vi "getConnectionPoints.vi"(0 "reference":refnum<class "SegmentedLineEdge.lvclass">, 5 "error in (no error)":errorcluster) -> (14 "reference out":refnum<class "SegmentedLineEdge.lvclass">, 15 "line":T1[](array[typedef]) {"y" format="%.2f"; "x" format="%.2f"}, 19 "error out":errorcluster)   [LabVIEW 2016, in "SegmentedLineEdge.lvclass"]
doc: "public Line2D getConnectionPoints()"
uses:
  <resource>/Framework/Providers/Open_GDS/UML/SegmentedLineEdge_class/SegmentedLineEdge.lvclass
  <resource>/Framework/Providers/Open_GDS/UML/General/Point/Point Point2D.ctl
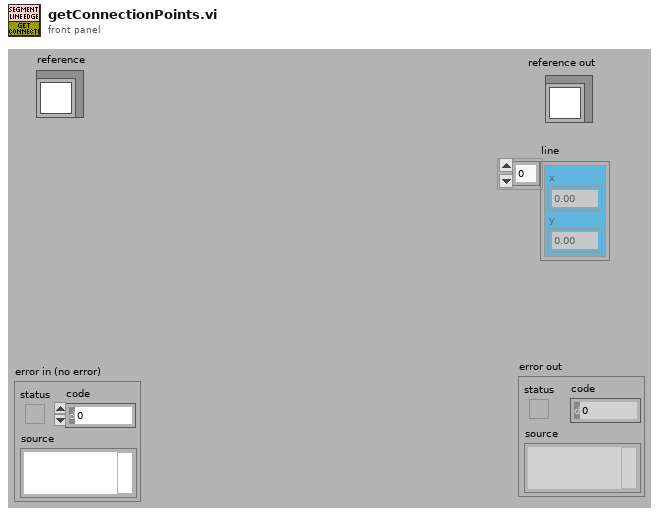
[diagram p1: front panel]
types:
  T1 = typedef "Point Point2D.ctl" = cluster{"x":dbl, "y":dbl}
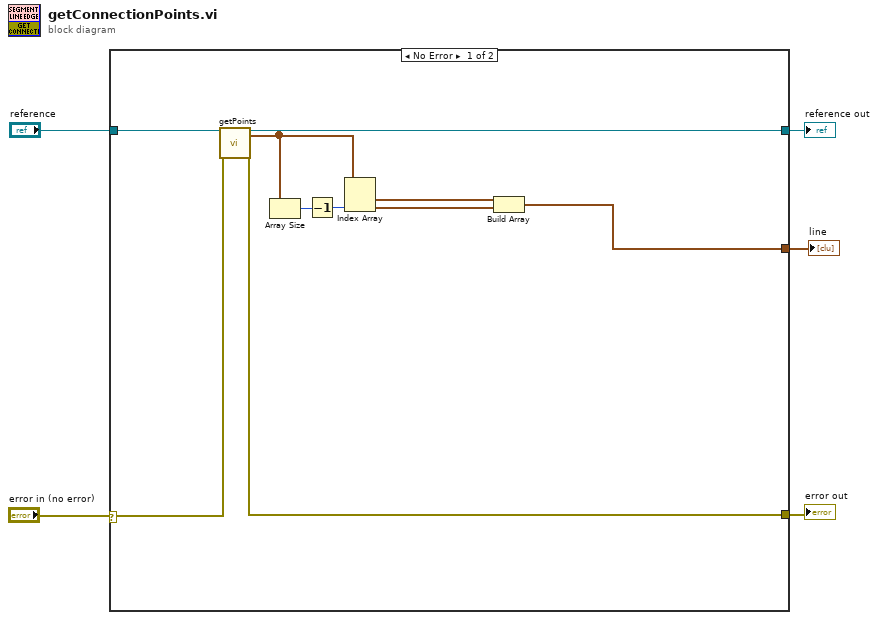
[diagram p0: block diagram]
diagram:
  n1 = case shown="No Error" "error in (no error)" {
    selector: "error in (no error)" -> [w6 w16]
    tunnel: "reference" -> [w15 w17]
    tunnel: [w14 w16] -> w4
    tunnel: [w13 w17] -> w3
    tunnel: [w12 _] -> w1
    frame No Error {
      n2 = call-dynamic "getPoints.vi"("reference"=w15, "error in (no error)"=w6) -> ("reference out"=w13:refnum<class "SegmentedLineEdge.lvclass">, "points"=w10:T1[], "error out"=w14:errorcluster)  [unwired: 15 in]
      n3 = Array Size(array=w10) -> (size(s)=w9:i32)
      n4 = Decrement(x=w9) -> (x-1=w8:i32)
      n5 = Index Array(array=w10, index #2=w8) -> (element #1=w11:T1, element #2=w7:T1)  [unwired: 1 in]
      n6 = Build Array(w11, w7) -> (w12:T1[])
    }
    frame Error {
    }
  }
  "reference out" <- w3
  "error out" <- w4
  "line" <- w1
